vi "Pico Status Code to String.vi"(1 "PICO_STATUS":u32) -> (0 "PICO_STATUS":string)   [LabVIEW 2016, in "pl1000.lvlib"]
uses:
  pl1000.lvlib
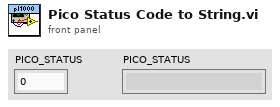
[diagram p1: front panel]
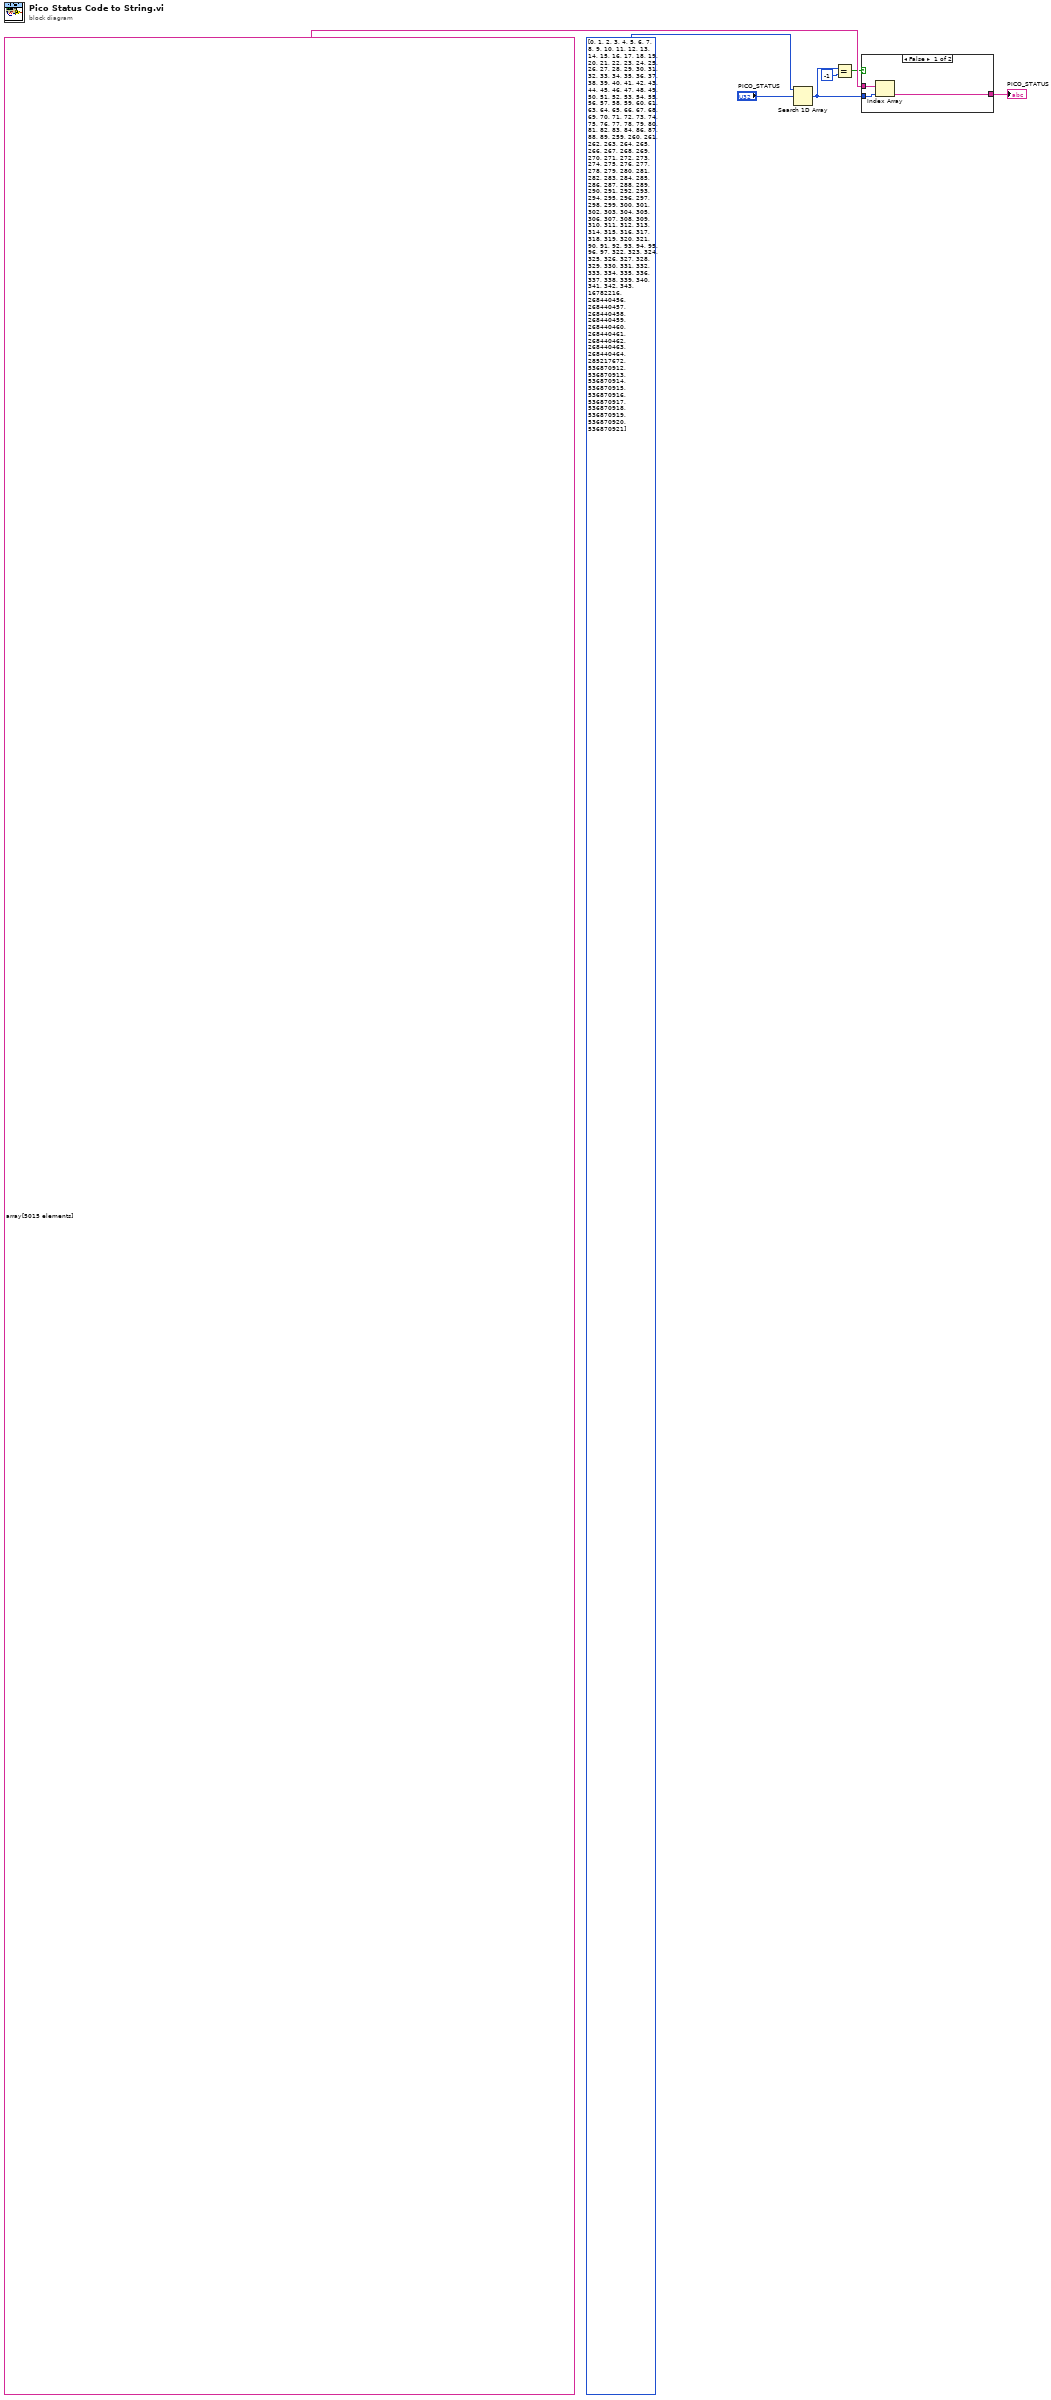
[diagram p0: block diagram]
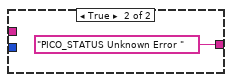
[diagram p2: hidden frame]
diagram:
  n1 = Search 1D Array(1D array=u32[] [0, 1, 2, 3, 4, 5, 6, 7, 8, 9, 10, 11, 12, 13, 14, 15, 16, 17, 18, 19, 20, 21, 22, 23, 24, 25, 26, 27, 28, 29, 30, 31, 32, 33, 34, 35, 36, 37, 38, 39, 40, 41, 42, 43, 44, 45, 46, 47, 48, 49, 50, 51, 52, 53, 54, 55, 56, 57, 58, 59, 60, 61, 63, 64, 65, 66, 67, 68, 69, 70, 71, 72, 73, 74, 75, 76, 77, 78, 79, 80, 81, 82, 83, 84, 86, 87, 88, 89, 259, 260, 261, 262, 263, 264, 265, 266, 267, 268, 269, 270, 271, 272, 273, 274, 275, 276, 277, 278, 279, 280, 281, 282, 283, 284, 285, 286, 287, 288, 289, 290, 291, 292, 293, 294, 295, 296, 297, 298, 299, 300, 301, 302, 303, 304, 305, 306, 307, 308, 309, 310, 311, 312, 313, 314, 315, 316, 317, 318, 319, 320, 321, 90, 91, 92, 93, 94, 95, 96, 97, 322, 323, 324, 325, 326, 327, 328, 329, 330, 331, 332, 333, 334, 335, 336, 337, 338, 339, 340, 341, 342, 343, 16782216, 268440456, 268440457, 268440458, 268440459, 268440460, 268440461, 268440462, 268440463, 268440464, 285217672, 536870912, 536870913, 536870914, 536870915, 536870916, 536870917, 536870918, 536870919, 536870920, 536870921] ("[user-defined codes]"), element="PICO_STATUS") -> (index of element=w3:i32)  [unwired: 1 in]
  n2 = Equal?(x=w3, y=-1) -> (x = y?=w4:bool)
  n3 = case shown="False" w4 {
    tunnel: string[] array[5015 elements] ("[user-defined descriptions]") -> [w10 _]
    tunnel: w3 -> [w9 _]
    tunnel: [w8 "PICO_STATUS Unknown Error " ("string")] -> w7
    frame False {
      n4 = Index Array(array=w10, index=w9) -> (element=w8:string)
    }
    frame True {
    }
  }
  "PICO_STATUS" <- w7
